vi "P5.vi"() -> ()   [LabVIEW 2024]
panel:
  in  "Numeric":dbl
  out "Heating":bool
  out "Cooling":bool
  in  "stop":bool
  in  "COMM_Name":refnum<visa-resource-name>
  out "Temp, C":dbl(slide) scale=0.0..100.0 scale format="%#1.3f"
  out "Scc, V":dbl(knob) scale=0.0..10.0 scale format="%#1.3f"
  out "AtoD, Hex":i32 format="%1x"
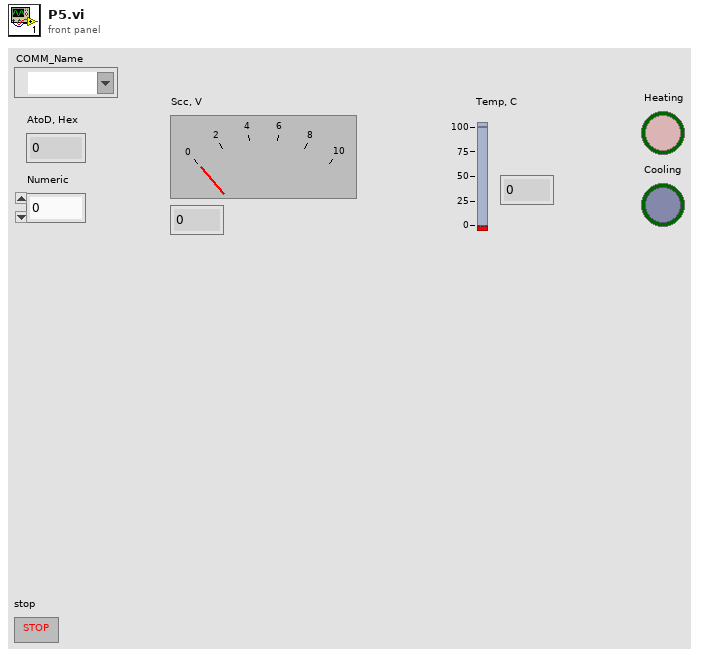
[diagram p1: front panel]
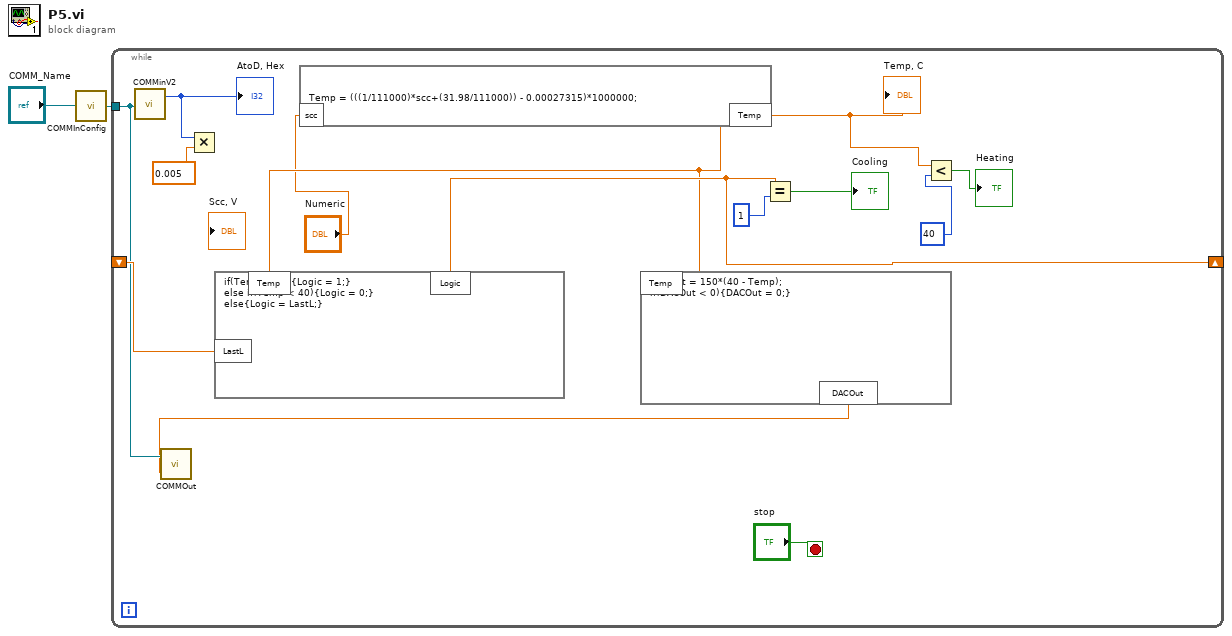
[diagram p0: block diagram]
diagram:
  n1 = call "COMMInConfig.vi"("COMM_in"="COMM_Name") -> ("COMM_Name"=w1:refnum<visa-resource-name>)
  n2 = while {
    tunnel: w1 -> [w8]
    shift-right: [w10] -> _
    shift-left: _ -> [w12]
    stop <- "stop" stop-if-true
    n3 = call "COMMinV2.vi"("VISA resource name"=w8) -> ("AtoDOut"=w15:i16)  [unwired: 1 out]
    "AtoD, Hex" <- w15
    n4 = Multiply(x=w15, y=0.005) -> ()  [unwired: 1 out]
    n5 = formula code="Temp = (((1/111000)*scc+(31.98/111000)) - 0.00027315)*1000000;"("scc"="Numeric") -> ("Temp"=w6:dbl)
    "Temp, C" <- w6
    n6 = formula code="if(Temp > 41){Logic = 1;}\nelse if(Temp < 40){Logic = 0;}\nelse{Logic = LastL;}"("Temp"=w6, "LastL"=w12) -> ("Logic"=w10:dbl)
    n7 = formula code="DACOut = 150*(40 - Temp);\nif(DACOut < 0){DACOut = 0;}"("Temp"=w6) -> ("DACOut"=w7:dbl)
    n8 = call "COMMOut.vi"("Numeric"=w7, "VISA resource name"=w8) -> ()
    n9 = Equal?(x=w10, y=1) -> (x = y?=→"Cooling":bool)
    n10 = Less?(x=w6, y=40) -> (x < y?=→"Heating":bool)
  }
